vi "Set Working Mode.vi"(6 "Prioritize Data?":bool, 8 "error in":errorcluster, 9 "Data":variant, 10 "Message":string) -> (0 "error out":errorcluster)   [LabVIEW 2024, in "Tester Working Mode.lvlib"]
uses:
  Tester Working Mode.lvlib
  Tester Internal Communication/QMH Item.ctl
  Tester Internal Communication/Queues - Get.vi
  Tester Internal Communication/Tester InterComm.lvlib
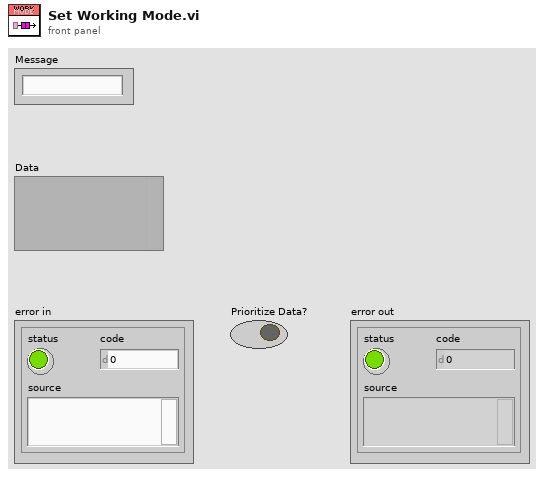
[diagram p1: front panel]
types:
  T1 = typedef "Tester InterComm.lvlib/QMH Item.ctl" = cluster{"Message":string, "Data":variant}
  T2 = typedef "Tester InterComm.lvlib/Process Queues.ctl" = cluster{"UI":refnum<queue>, "Working Mode":refnum<queue>}
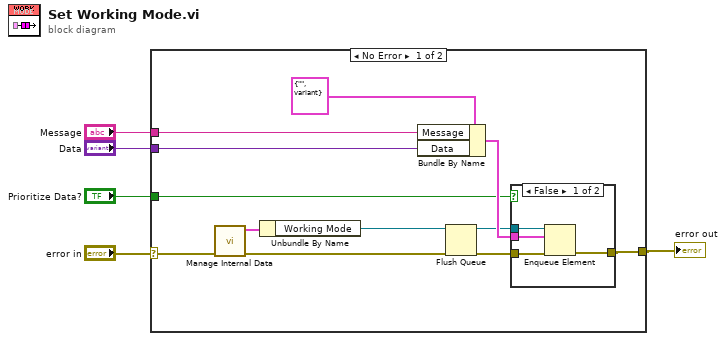
[diagram p0: block diagram]
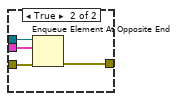
[diagram p2: hidden frame]
diagram:
  n1 = case shown="No Error" "error in" {
    selector: "error in" -> [w11 w26]
    tunnel: "Message" -> [w15 _]
    tunnel: "Data" -> [w14 _]
    tunnel: "Prioritize Data?" -> [w12 _]
    tunnel: [w10 w26] -> w1
    frame No Error {
      n2 = call-poly "Manage Internal Data.vi"("error in"=w11) -> ("error out"=w6:errorcluster, "Queues Out"=w17:T2)  [unwired: 9 in]
      n3 = Unbundle By Name(w17) -> ("Working Mode"=w7:refnum<queue>)
      n4 = Bundle By Name(cluster=T1 {"Message"="", "Data"=variant} ("element"), "Message"=w15, "Data"=w14) -> (w13:T1)
      n5 = Flush Queue(queue=w7, error in (no error)=w6) -> (queue out=w9:refnum<queue>, error out=w8:errorcluster)  [unwired: 1 out]
      n6 = case shown="False" w12 {
        tunnel: w9 -> [w21 w23]
        tunnel: w8 -> [w20 w25]
        tunnel: w13 -> [w19 w24]
        tunnel: [w18 w22] -> w10
        frame False {
          n7 = Enqueue Element(queue=w21, element=w19, error in (no error)=w20) -> (error out=w18:errorcluster)  [unwired: 1 in, 2 out]
        }
        frame True {
          n8 = Enqueue Element At Opposite End(queue=w23, element=w24, error in (no error)=w25) -> (error out=w22:errorcluster)  [unwired: 1 in, 2 out]
        }
      }
    }
    frame Error {
    }
  }
  "error out" <- w1
